vi "ProcessLidarData.vi"(0 "WhatAroundMe?MM":cluster{"T":dbl, "Range":dbl, "Bearing":dbl}[](array[cluster])) -> (1 "Collision":bool, 2 "data array [mag, phase (deg)]":cluster{"magnitude":dbl, "phase":dbl}[](array[cluster]))   [LabVIEW 2012]
doc: "Strips time cell out of LIDAR array data"
panel:
  # "This subVI just strips off \nthe time data so that \nLIDAR data can be polar \nplotted."
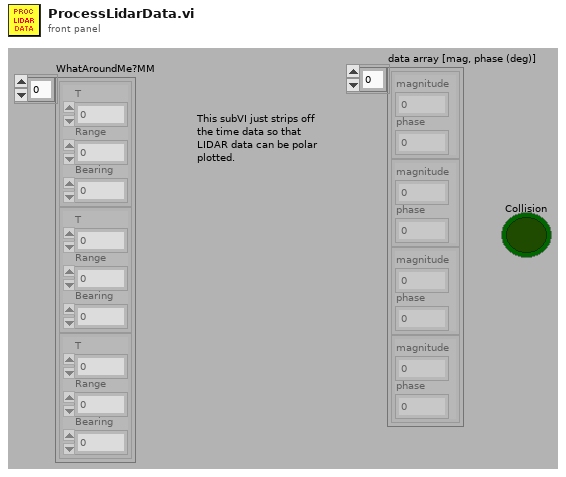
[diagram p1: front panel]
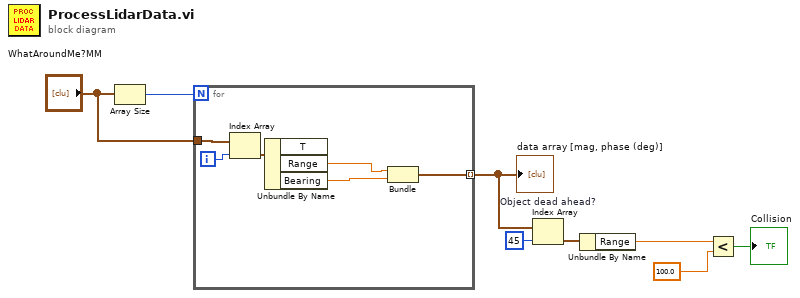
[diagram p0: block diagram]
diagram:
  n1 = Array Size(array="WhatAroundMe?MM") -> (size(s)=w8:i32)
  n2 = for {
    N: w8 -> [_]
    tunnel: "WhatAroundMe?MM" -> [w14]
    tunnel: [w9] -> w4 mode=indexing
    i -> [w13]
    n3 = Index Array "Index Array"(array=w14, index=w13) -> (element=w12:cluster{"T":dbl, "Range":dbl, "Bearing":dbl})
    n4 = Unbundle By Name "Unbundle By Name"(w12) -> ("Range"=w11:dbl, "Bearing"=w10:dbl)  [unwired: 1 out]
    n5 = Bundle "Bundle"("Range"=w11, "Bearing"=w10) -> (w9:cluster{"Range":dbl, "Bearing":dbl})  [unwired: 1 in]
  }
  "data array [mag, phase (deg)]" <- w4
  n6 = Index Array "Object dead ahead?"(array=w4, index=45) -> (element=w3:cluster{"Range":dbl, "Bearing":dbl})
  n7 = Unbundle By Name(w3) -> ("Range"=w2:dbl)
  n8 = Less?(x=w2, y=100.0) -> (x < y?=→"Collision":bool)
